vi "Enable Remote Sensing.vi"(8 "error in (no error)":errorcluster, 10 "Enable Remote Sensing (T: Enable)":bool=TRUE, 11 "VISA resource name":refnum<visa-resource-name>) -> (0 "error out":errorcluster, 3 "VISA resource name out":refnum<visa-resource-name>)   [LabVIEW 2019, in "Keithley 24XX.lvlib"]
doc: "Enables Remote (4-wire) sensing. This type of sensing allows the instrument to bypass the input and output leads and make a more accurate measurement at the device under test. This also allows the source to adjust its voltage so that the desired voltage is located at the sensing leads, not at the input and output jacks."
uses:
  Keithley 24XX.lvlib
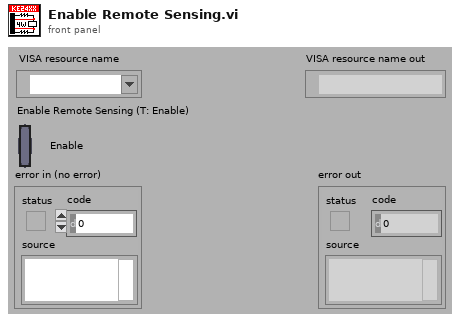
[diagram p1: front panel]
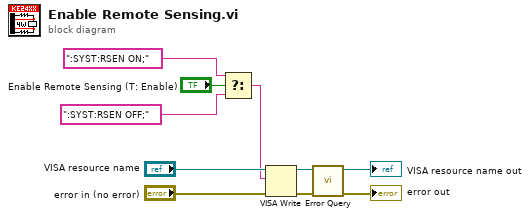
[diagram p0: block diagram]
diagram:
  n1 = Select(t=":SYST:RSEN ON;", s="Enable Remote Sensing (T: Enable)", f=":SYST:RSEN OFF;") -> (s? t:f=w1:string)
  n2 = VISA Write(VISA resource name="VISA resource name", write buffer=w1, error in (no error)="error in (no error)") -> (VISA resource name out=w6:refnum<visa-resource-name>, error out=w5:errorcluster)  [unwired: 1 out]
  n3 = call "Error Query.vi"("error in (no error)"=w5, "VISA resource name"=w6) -> ("error out"=→"error out":errorcluster, "VISA resource name out"=→"VISA resource name out":refnum<visa-resource-name>)  [unwired: 6 in, 2 out]
